vi "ReadWriteUserInfoData.vi"(0 "User Info  Array In":T1[](array[typedef]) {"UserType" items=["Admin", "Operator"]}, 11 "Error in (no error)":errorcluster, 13 "Operation":enum16{"Write", "Read"}(ring)=enum."Read") -> (4 "User Info Array of Clusters Out":T1[](array[typedef]) {"UserType" items=["Admin", "Operator"]}, 6 "User Info Array out":string[][](array[string]), 15 "Error out":errorcluster)   [LabVIEW 2021]
uses:
  Controls/UserTypes.ctl
  Controls/UserInfo.ctl
panel:
  out "Password":string
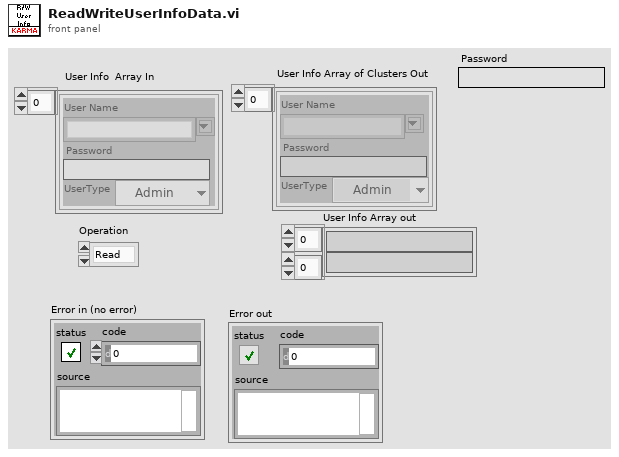
[diagram p1: front panel]
types:
  T1 = typedef "UserInfo.ctl" = cluster{"User Name":string, "Password":string, "UserType":T2}
  T2 = typedef "UserTypes.ctl" = u16
  T3 = typedef "Paths.ctl" = cluster{"Configuration":path, "Event Logs":path, "Error Logs":path, "Macros":path, "Camera Settings":path, "Settings.ini":path, "UserInfo.bin":path, "TimeStamp File":path, "FileCounter.txt":path, "FFC Images":path, "Calibration.txt":path, "Bright Images - FFC":path, "Dark Images - FFC":path, "Last FFC Time File":path, "BG Subtraction Folder":path, "BG Mask":path, "LUTs Folder":path}
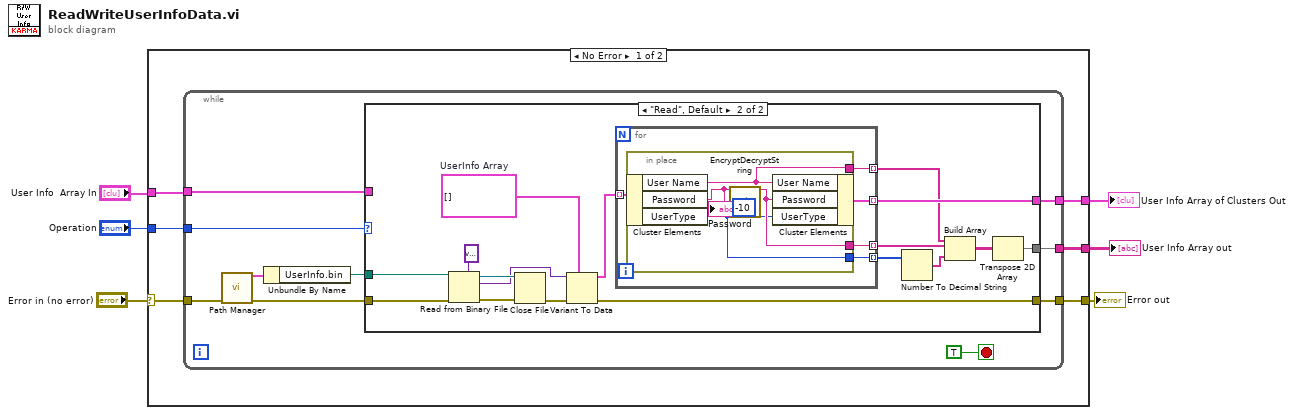
[diagram p0: block diagram]
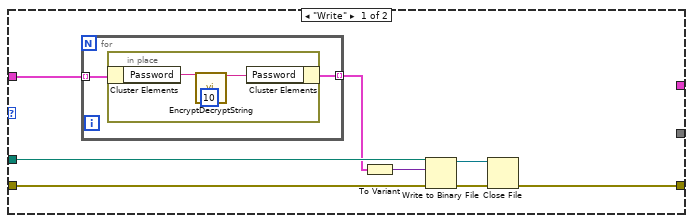
[diagram p2: hidden frame]
diagram:
  n1 = case shown="No Error" "Error in (no error)" {
    selector: "Error in (no error)" -> [w11 w63]
    tunnel: "Operation" -> [w12 _]
    tunnel: [w10 w63] -> w4
    tunnel: "User Info  Array In" -> [w9 _]
    tunnel: [w8 _] -> w2
    tunnel: [w7 _] -> w1
    frame No Error {
      n2 = while {
        tunnel: w12 -> [w22]
        tunnel: w11 -> [w19]
        tunnel: [w17] -> w10
        tunnel: w9 -> [w16]
        tunnel: [w15] -> w8
        tunnel: [w13] -> w7
        stop <- TRUE stop-if-true
        n3 = call "Path Manager.vi"("error in (no error)"=w19) -> ("Cluster"=w21:T3, "Error out"=w18:errorcluster)  [unwired: 13 in]
        n4 = Unbundle By Name(w21) -> ("UserInfo.bin"=w20:path)
        n5 = case shown="\"Read\", Default" w22 {
          tunnel: w20 -> [w30 w46]
          tunnel: w18 -> [w29 w47]
          tunnel: [w25 w48] -> w17
          tunnel: w16 -> [w24 _]
          tunnel: [_ w39] -> w15
          tunnel: [_ w41] -> w13
          frame "Write" {
            n6 = for {
              tunnel: w24 -> [w32] mode=indexing
              tunnel: [w31] -> w23 mode=indexing
              n7 = in-place {
                n8 = in-place-cluster #1(w32) -> ("Password"=w35:string)
                n9 = call "EncryptDecryptString.vi"("Original"=w35, "ROT by..."=10) -> ("ROT'd string"=w34:string)  [unwired: 13 in]
                n10 = in-place-cluster #1("Password"=w34) -> (w31:T1)
              }
            }
            n11 = To Variant(anything=w23) -> (Variant=w28:variant)
            n12 = Write to Binary File(file (use dialog)=w30, data=w28, error in=w29) -> (refnum out=w27:refnum<file>, error out=w26:errorcluster)  [unwired: 3 in, 1 out]
            n13 = Close File(refnum=w27, error in=w26) -> (error out=w25:errorcluster)  [unwired: 1 out]
          }
          frame "Read", Default {
            w44 = T1[] []  # UserInfo Array
            n14 = Read from Binary File(5:variant, 8:w47, 11:w46) -> (0:w51:errorcluster, 2:w45:variant, 3:w50:refnum<file>)  [unwired: 3 in, 1 out]
            n15 = Close File(refnum=w50, error in=w51) -> (error out=w49:errorcluster)  [unwired: 1 out]
            n16 = Variant To Data(error in=w49, type=w44, Variant=w45) -> (data=w40:T1[], error out=w48:errorcluster)
            n17 = for {
              tunnel: w40 -> [w57] mode=indexing
              tunnel: [w56] -> w39 mode=indexing
              tunnel: [w55] -> w38 mode=indexing
              tunnel: [w54] -> w36 mode=indexing
              tunnel: [w53] -> w37 mode=indexing
              n18 = in-place {
                in-place-border: [w60] -> w53
                in-place-border: [w59] -> w55
                in-place-border: [w58] -> w54
                n19 = in-place-cluster #2(w57) -> ("User Name"=w59:string, "Password"=w61:string, "UserType"=w58:T2)
                "Password" <- w61
                n20 = call "EncryptDecryptString.vi"("Original"=w61, "ROT by..."=-10) -> ("ROT'd string"=w60:string)  [unwired: 13 in]
                n21 = in-place-cluster #2("User Name"=w59, "Password"=w60, "UserType"=w58) -> (w56:T1)
              }
            }
            n22 = Number To Decimal String(number=w36) -> (decimal integer string=w43:string[])  [unwired: 1 in]
            n23 = Build Array(w38, w37, w43) -> (w42:string[][])
            n24 = Transpose 2D Array(2D array=w42) -> (transposed array=w41:string[][])
          }
        }
      }
    }
    frame Error {
    }
  }
  "Error out" <- w4
  "User Info Array of Clusters Out" <- w2
  "User Info Array out" <- w1
